vi "Choreo_TrajectoryState_FieldWidth.vi"() -> (3 "Field_Width_Meters":dbl)   [LabVIEW 2019]
doc: "Return FRC field width. This is valid for the current game only.\n\nInputs:\n <none>\n\nOutputs: \n - Field_Width_Meters - double - Playing field width. meters"
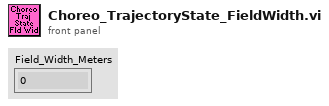
[diagram p1: front panel]
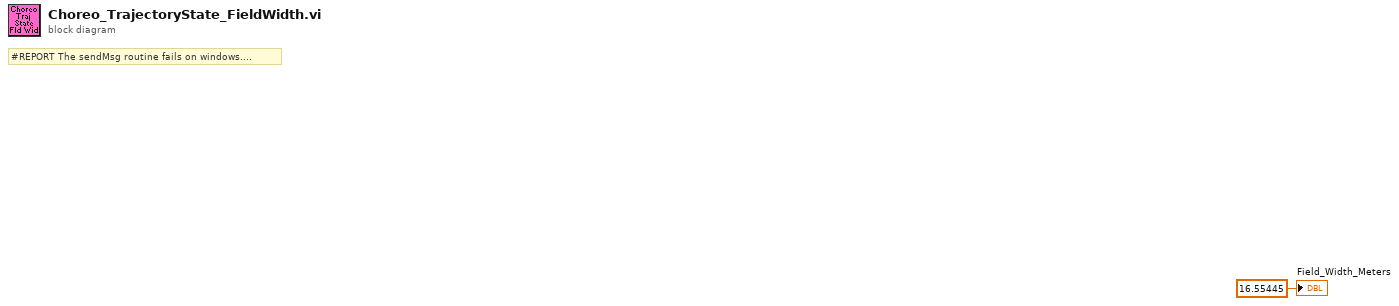
[diagram p0: block diagram]
diagram:
  # "#REPORT The sendMsg routine fails on windows...."
  "Field_Width_Meters" <- 16.55445 ("Field_Width_Meters")
